vi "Unflat JSON.vi"(8 "error in (no error)":errorcluster, 11 "File interpreter in":refnum<class "File interpreter.lvclass">) -> (0 "error out":errorcluster, 2 "value":T1, 3 "File interpreter out":refnum<class "File interpreter.lvclass">)   [LabVIEW 2018, in "File interpreter.lvclass"]
uses:
  File interpreter.lvclass
  File interpreter.lvclass/File interpreter.ctl
  JSON reader/JSON reader.lvclass
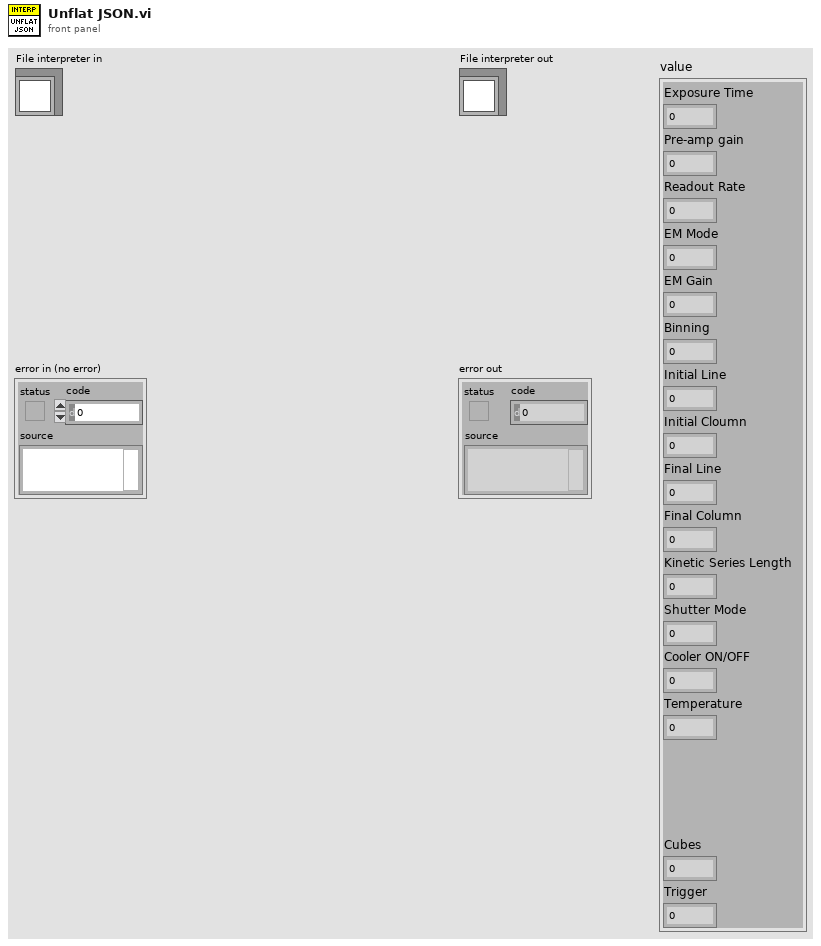
[diagram p1: front panel]
types:
  T1 = cluster{"Exposure Time":sgl, "Pre-amp gain":u8, "Readout Rate":u8, "EM Mode":u8, "EM Gain":u16, "Binning":u16, "Initial Line":u16, "Initial Cloumn":u16, "Final Line":u16, "Final Column":u16, "Kinetic Series Length":u32, "Shutter Mode":u8, "Cooler ON/OFF":u16, "Temperature":i8, "Cubes":u32, "Trigger":u16}
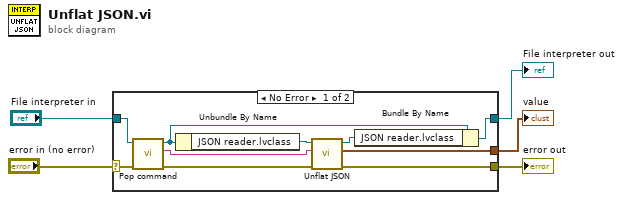
[diagram p0: block diagram]
diagram:
  n1 = case shown="No Error" "error in (no error)" {
    selector: "error in (no error)" -> [w15 w17]
    tunnel: [w7 w17] -> w4
    tunnel: [w6 w16] -> w2
    tunnel: "File interpreter in" -> [w14 w16]
    tunnel: [w10 _] -> w1
    frame No Error {
      n2 = call "Pop command.vi"("error in (no error)"=w15, "File interpreter in"=w14) -> ("error out"=w11:errorcluster, "command"=w12:string, "File interpreter out"=w9:refnum<class "File interpreter.lvclass">)  [unwired: 7 in]
      n3 = Unbundle By Name(w9) -> ("JSON reader.lvclass"=w13:refnum<class "JSON reader.lvclass">)
      n4 = call "Unflat JSON.vi"("error in (no error)"=w11, "JSON string"=w12, "JSON reader in"=w13) -> ("error out"=w7:errorcluster, "value"=w10:T1, "JSON reader out"=w8:refnum<class "JSON reader.lvclass">)  [unwired: 6 in]
      n5 = Bundle By Name(cluster=w9, "JSON reader.lvclass"=w8) -> (w6:refnum<class "File interpreter.lvclass">)
    }
    frame Error {
    }
  }
  "error out" <- w4
  "File interpreter out" <- w2
  "value" <- w1
